vi "Write Initialized Status (Array).vi"(8 "error in":errorcluster, 10 "Initialized":bool[](array[boolean]), 11 "Cycler in":refnum<class "Cycler.lvclass">) -> (0 "error out":errorcluster, 3 "Cycler out":refnum<class "Cycler.lvclass">)   [LabVIEW 2023, in "Cycler.lvclass"]
uses:
  Cycler.lvclass
  Cycler.lvclass/Cycler.ctl
  <vilib>/ADAS Replay HIL/Channels/Tag Wrapper/Polymorphic/Write Channel (Boolean).vi
  <vilib>/ADAS Replay HIL/Channels/Tag Wrapper/Polymorphic/Write Channel (Boolean).vi/cccb8e89-591f-4bb4-9d4e-ae06ba1f5498.vi
  <vilib>/ADAS Replay HIL/Channels/Tag Wrapper/Polymorphic/Write Channel (Boolean).vi/cccb8e89-591f-4bb4-9d4e-ae06ba1f5498.vi/4bc1c15b-36ab-481f-b8dd-c64075ce723a.vi
  <vilib>/ADAS Replay HIL/Channels/Tag Wrapper/Polymorphic/Write Channel (Boolean).vi/cccb8e89-591f-4bb4-9d4e-ae06ba1f5498.vi/d83cb72b-7713-41fc-a3d1-682de79cf574.vi
  <vilib>/ADAS Replay HIL/Channels/Tag Wrapper/Tag Wrapper.lvlib
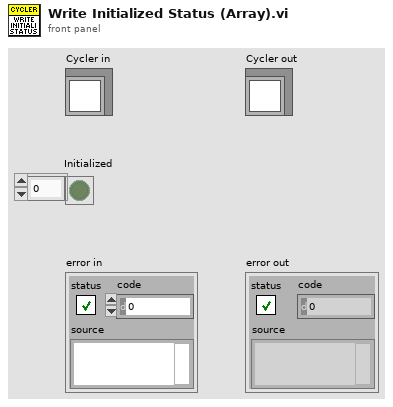
[diagram p1: front panel]
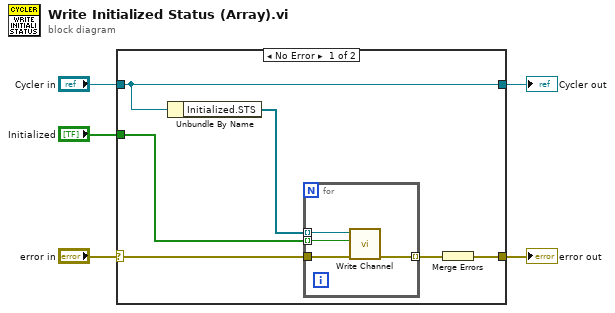
[diagram p0: block diagram]
diagram:
  n1 = case shown="No Error" "error in" {
    selector: "error in" -> [w11 w16]
    tunnel: [w6 w16] -> w4
    tunnel: [w8 w17] -> w2
    tunnel: "Cycler in" -> [w8 w17]
    tunnel: "Initialized" -> [w9 _]
    frame No Error {
      n2 = Unbundle By Name(w8) -> ("Initialized.STS"=w7:refnum<k21>[])
      n3 = for {
        tunnel: w9 -> [w13] mode=indexing
        tunnel: w7 -> [w12] mode=indexing
        tunnel: w11 -> [w15]
        tunnel: [w14] -> w10 mode=indexing
        n4 = call-poly <vilib>:"Write Channel.vi"("error in"=w15, "Value to Write"=w13, "ADAS HIL Channel in"=w12) -> ("error out"=w14:errorcluster)  [unwired: 6 in, 2 out]
      }
      n5 = Merge Errors(w10) -> (w6:errorcluster)
    }
    frame Error {
    }
  }
  "error out" <- w4
  "Cycler out" <- w2
